vi "Semaphore Open.vi"(6 "mode":u32, 7 "value":u32, 8 "error in (no error)":errorcluster, 9 "oflag":u32, 10 "name":string, 11 "Semaphore in":T1) -> (0 "error out":errorcluster, 2 "semaphore ptr out":u64, 3 "Semaphore out":T1)   [LabVIEW 2013, in "Linux RT IPC.POSIX Threads.lvlib" / "Semaphore.lvclass"]
doc: "Calls sem_open() to open a reference to a named semaphore and returns a pointer.\n\nThis VI initializes the semaphore object and sets its default values.\n\nRefer to online POSIX documentation for more information."
uses:
  <vilib>/NI/NI Linux RT IPC/POSIX Threads/Classes/Semaphore/Semaphore.lvclass
  <vilib>/NI/NI Linux RT IPC/POSIX Threads/Classes/POSIX Thread Object/POSIX Thread Object.lvclass
  <vilib>/NI/NI Linux RT IPC/POSIX Threads/Classes/Semaphore/Controls/reference.ctl
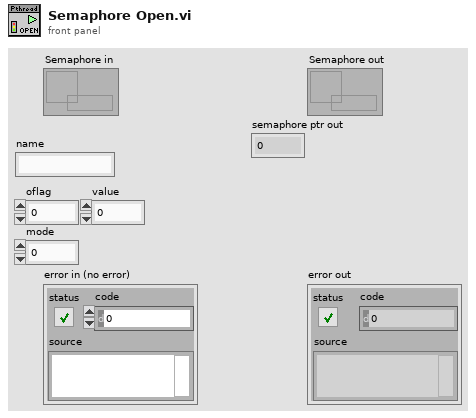
[diagram p1: front panel]
types:
  T1 = typedef "Linux RT IPC.POSIX Threads.lvlib/Semaphore.lvclass/reference.ctl" = refnum<data-value>
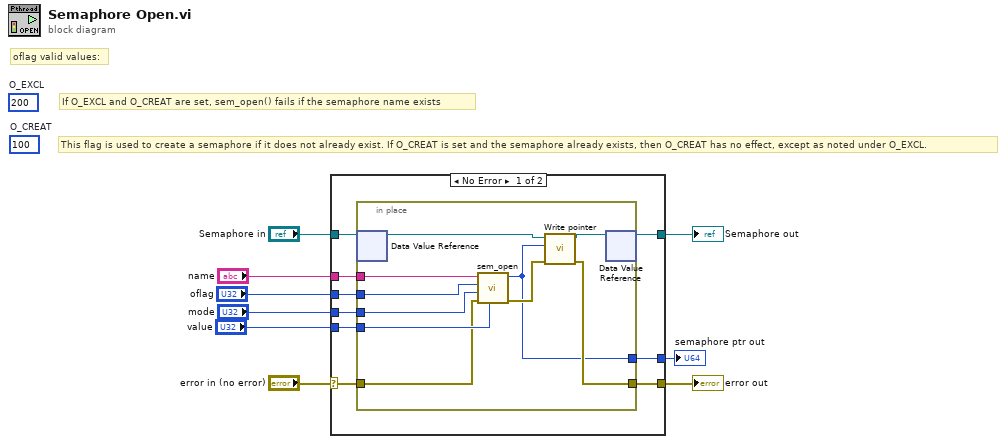
[diagram p0: block diagram]
diagram:
  (unwired) u32 200  # O_EXCL
  (unwired) u32 100  # O_CREAT
  # "If O_EXCL and O_CREAT are set, sem_open() fails if the semaphore name exists"
  # "This flag is used to create a semaphore if it does not already exist. If O_CREAT is set and the semaphore already exists, then O_CREAT has no effect, except as noted under O_EXCL."
  # "oflag valid values:"
  n1 = case shown="No Error" "error in (no error)" {
    selector: "error in (no error)" -> [w11 w29]
    tunnel: "Semaphore in" -> [w18 w30]
    tunnel: [w17 w30] -> w6
    tunnel: [w16 w29] -> w7
    tunnel: "name" -> [w15 _]
    tunnel: "oflag" -> [w14 _]
    tunnel: "mode" -> [w13 _]
    tunnel: "value" -> [w12 _]
    tunnel: [w10 _] -> w1
    frame No Error {
      n2 = in-place {
        in-place-border: [w20] -> w16
        in-place-border: w15 -> [w28]
        in-place-border: w14 -> [w27]
        in-place-border: w13 -> [w26]
        in-place-border: w12 -> [w25]
        in-place-border: w11 -> [w24]
        in-place-border: [w19] -> w10
        n3 = in-place-dvr #1(w18) -> (w23:refnum<class "Semaphore.lvclass">)  [unwired: 1 out]
        n4 = call <vilib>:"sem_open.vi"("value"=w25, "error in (no error)"=w24, "mode"=w26, "oflag"=w27, "name"=w28) -> ("error out"=w21:errorcluster, "semaphore ptr out"=w19:u64)  [unwired: 5 in]
        n5 = call <vilib>:"Write pointer.vi"("error in (no error)"=w21, "pointer"=w19, "POSIX Thread Object in"=w23) -> ("error out"=w20:errorcluster, "POSIX Thread Object out"=w22:refnum<class "Semaphore.lvclass">)  [unwired: 7 in]
        n6 = in-place-dvr #1(w22) -> (w17:T1)  [unwired: 1 out]
      }
    }
    frame Error {
    }
  }
  "error out" <- w7
  "Semaphore out" <- w6
  "semaphore ptr out" <- w1
